vi "Read Limit Test Result.vi"(0 "VISA resource name":refnum<visa-resource-name>, 5 "Limit Line (1)":i32=1 min=1 max=6, 11 "error in (no error)":errorcluster) -> (4 "VISA resource name out":refnum<visa-resource-name>, 6 "Judgement":i32(ring) items=["PASS"=0, "FAIL"=1, "ERROR"=-999], 15 "error out":errorcluster)   [LabVIEW 2020, in "Anritsu Signal Analyzer Series.lvlib"]
doc: "Queries Pass/Fail judgment and displays the result."
uses:
  Anritsu Signal Analyzer Series.lvlib
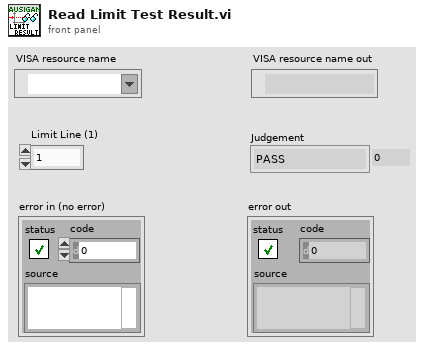
[diagram p1: front panel]
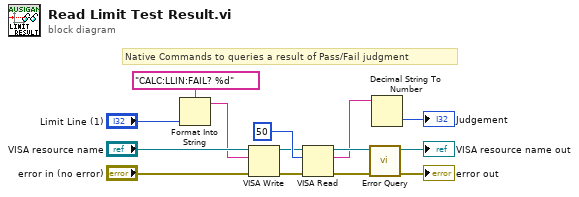
[diagram p0: block diagram]
diagram:
  # "Native Commands to queries a result of Pass/Fail judgment"
  n1 = Format Into String(format string="CALC:LLIN:FAIL? %d", "Limit Line (1)") -> (resulting string=w1:string)  [unwired: 2 in, 1 out]
  n2 = VISA Write(VISA resource name="VISA resource name", write buffer=w1, error in (no error)="error in (no error)") -> (VISA resource name out=w8:refnum<visa-resource-name>, error out=w9:errorcluster)  [unwired: 1 out]
  n3 = VISA Read(VISA resource name=w8, byte count=u32 50 ("byte count (0)"), error in (no error)=w9) -> (VISA resource name out=w7:refnum<visa-resource-name>, read buffer=w5:string, error out=w6:errorcluster)  [unwired: 1 out]
  n4 = call "Error Query.vi"("error in (no error)"=w6, "VISA resource name"=w7) -> ("error out"=→"error out":errorcluster, "VISA resource name out"=→"VISA resource name out":refnum<visa-resource-name>)  [unwired: 6 in, 2 out]
  n5 = Decimal String To Number(string=w5) -> (number=→"Judgement":i32)  [unwired: 2 in, 1 out]
